vi "Calibration_load_file.vi"(10 "DEV SN":u32) -> (2 "Calib value-mA":dbl, 3 "Calib value-uA":dbl)   [LabVIEW 2017]
uses:
  Range_Shunt_selector.ctl
  <vilib>/Utility/config.llb/Read Key (Double).vi
  <vilib>/Utility/config.llb/NI_LVConfig.lvlib
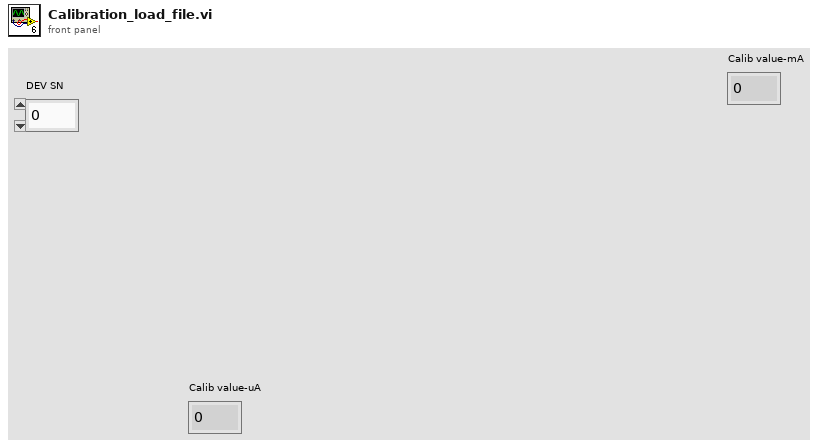
[diagram p1: front panel]
types:
  T1 = typedef "Range_Shunt_selector.ctl" = enum16{"uA Range  Rs = 3.3ohm", "mA Range Rs = 3.3ohm", "mA Range Rs = 1ohm", "mA Range Rs = 1ohm - X2"}
  T2 = typedef "NI_LVConfig.lvlib/Config Data RefNum.ctl" = refnum<k1>
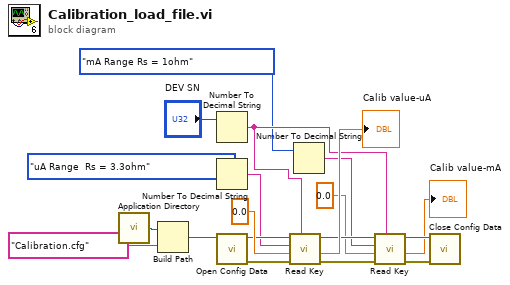
[diagram p0: block diagram]
diagram:
  n1 = call <vilib>:"Application Directory.vi"() -> ("Application Directory"=w19:path)
  n2 = Build Path(base path=w19, name or relative path="Calibration.cfg") -> (appended path=w17:path)
  n3 = Number To Decimal String(number="DEV SN") -> (decimal integer string=w7:string)  [unwired: 1 in]
  n4 = Number To Decimal String(number=Range_Shunt_selector."uA Range  Rs = 3.3ohm" ("Range - Shunts")) -> (decimal integer string=w10:string)  [unwired: 1 in]
  n5 = call <vilib>:"Open Config Data.vi"("configuration file path"=w17) -> ("error out"=w14:errorcluster, "refnum"=w15:T2)  [unwired: 8 in, 1 out]
  n6 = call-poly <vilib>:"Read Key.vi"("section"=w7, "error in (no error)"=w14, "default value"=0.0, "key"=w10, "refnum"=w15) -> ("error out"=w4:errorcluster, "value"=→"Calib value-uA":dbl, "refnum out"=w9:T2)  [unwired: 3 in, 1 out]
  n7 = Number To Decimal String(number=Range_Shunt_selector."mA Range Rs = 1ohm" ("Range - Shunts 2")) -> (decimal integer string=w5:string)  [unwired: 1 in]
  n8 = call-poly <vilib>:"Read Key.vi"("section"=w7, "error in (no error)"=w4, "default value"=0.0, "key"=w5, "refnum"=w9) -> ("error out"=w1:errorcluster, "value"=→"Calib value-mA":dbl, "refnum out"=w8:T2)  [unwired: 3 in, 1 out]
  n9 = call <vilib>:"Close Config Data.vi"("error in (no error)"=w1, "refnum"=w8) -> ()  [unwired: 8 in, 2 out]
